vi "IsDebug.vi"() -> (1 "Boolean":bool)   [LabVIEW 2014]
panel:
  out "call chain":string[](array[string])
  out "size(s)":i32
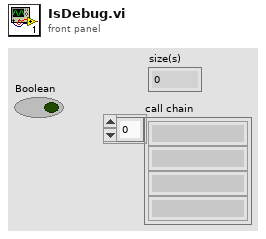
[diagram p1: front panel]
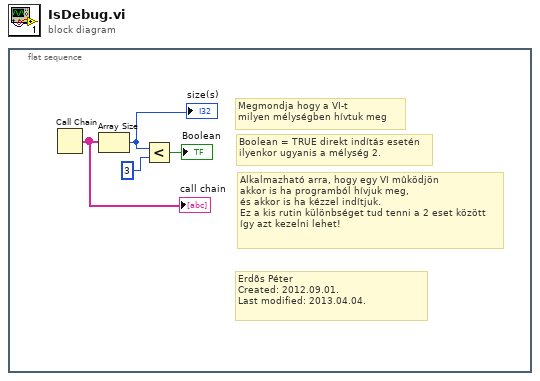
[diagram p0: block diagram]
diagram:
  n1 = flat-sequence {
    frame #0 {
      # "Alkalmazható arra, hogy egy VI mûködjön\nakkor is ha programból hívjuk meg,\nés akkor is ha kézzel indítjuk.\nEz a kis rutin különbséget tud tenni a 2 eset között\nígy azt kezelni lehet!"
      # "Boolean = TRUE direkt indítás esetén\nilyenkor ugyanis a mélység 2."
      # "Megmondja hogy a VI-t\nmilyen mélységben hívtuk meg"
      # "Erdõs Péter\nCreated: 2012.09.01.\nLast modified: 2013.04.04."
      n2 = Call Chain() -> (call chain=w1:string[])
      "call chain" <- w1
      n3 = Array Size(array=w1) -> (size(s)=w2:i32)
      "size(s)" <- w2
      n4 = Less?(x=w2, y=3) -> (x < y?=→"Boolean":bool)
    }
  }
